vi "CurrentMeterLoop.vi"(8 "Error In":errorcluster, 9 "ABLE Configuration":T1, 10 "Current Meter Data":refnum<notifier>, 11 "Current Meter Action Queue":refnum<queue>) -> (0 "Error Out":errorcluster)   [LabVIEW 2012]
uses:
  CurrentMeterQueueElement.ctl
  CurrentMeterAction.ctl
  ABLEConfiguration.ctl
  DisplayConfiguration.ctl
  FolderConfiguration.ctl
  AlarmsConfiguration.ctl
  Keithley6485Configuration.ctl
  Keithley6482Configuration.ctl
  CurrentMeterData.ctl
  <vilib>/Utility/error.llb/DialogType.ctl
  libs/LV-Utilities/LV-Utilities.lvlib
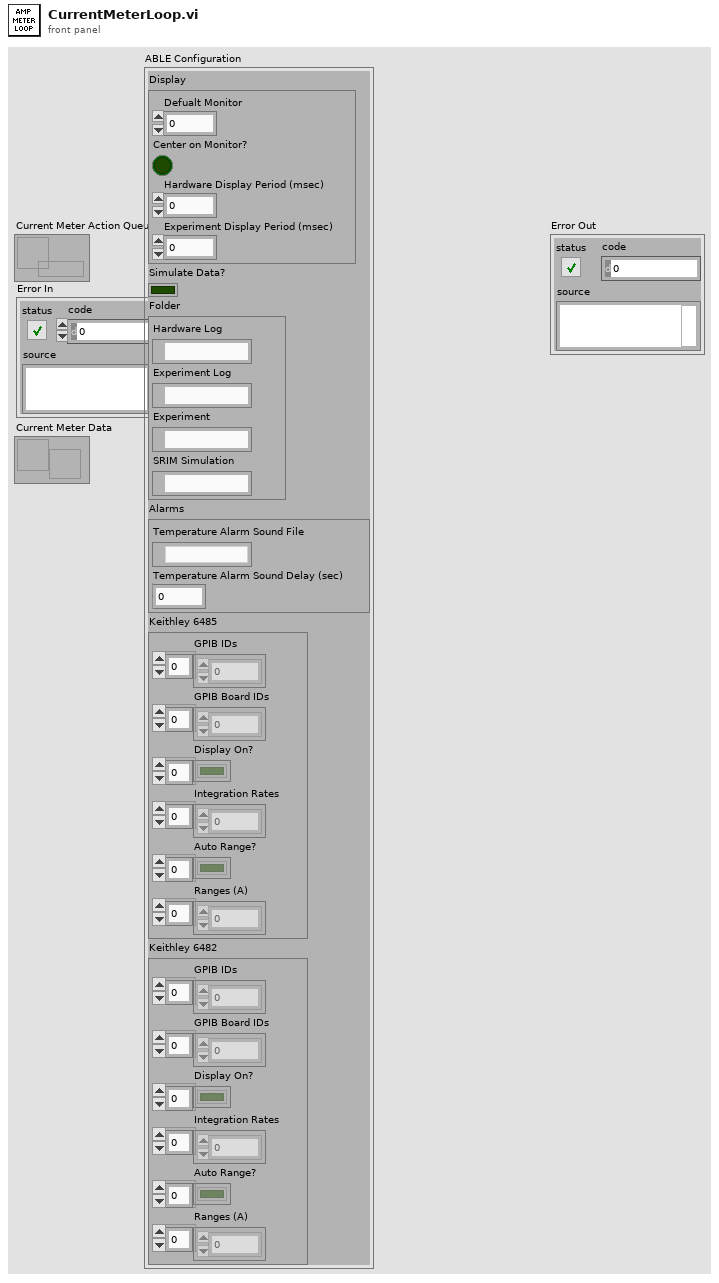
[diagram p1: front panel]
types:
  T1 = typedef "ABLEConfiguration.ctl" = cluster{"Display":T2, "Simulate Data?":bool, "Folder":T3, "Alarms":T4, "Keithley 6485":T5, "Keithley 6482":T6}
  T2 = typedef "DisplayConfiguration.ctl" = cluster{"Defualt Monitor":u16, "Center on Monitor?":bool, "Hardware Display Period (msec)":u32, "Experiment Display Period (msec)":u32}
  T3 = typedef "FolderConfiguration.ctl" = cluster{"Hardware Log":path, "Experiment Log":path, "Experiment":path, "SRIM Simulation":path}
  T4 = typedef "AlarmsConfiguration.ctl" = cluster{"Temperature Alarm Sound File":path, "Temperature Alarm Sound Delay (sec)":dbl}
  T5 = typedef "Keithley6485Configuration.ctl" = cluster{"GPIB IDs":u8[], "GPIB Board IDs":u8[], "Display On?":bool[], "Integration Rates":dbl[], "Auto Range?":bool[], "Ranges (A)":dbl[]}
  T6 = typedef "Keithley6482Configuration.ctl" = cluster{"GPIB IDs":u8[], "GPIB Board IDs":u8[], "Display On?":bool[], "Integration Rates":dbl[], "Auto Range?":bool[], "Ranges (A)":dbl[]}
  T7 = typedef "CurrentMeterData.ctl" = dbl[]
  T8 = typedef "CurrentMeterQueueElement.ctl" = cluster{"Action":T9, "Data":variant}
  T9 = typedef "CurrentMeterAction.ctl" = enum16{"Initialize", "Read", "Simulate", "Error", "Shutdown"}
  T10 = typedef "DialogType.ctl" = u16
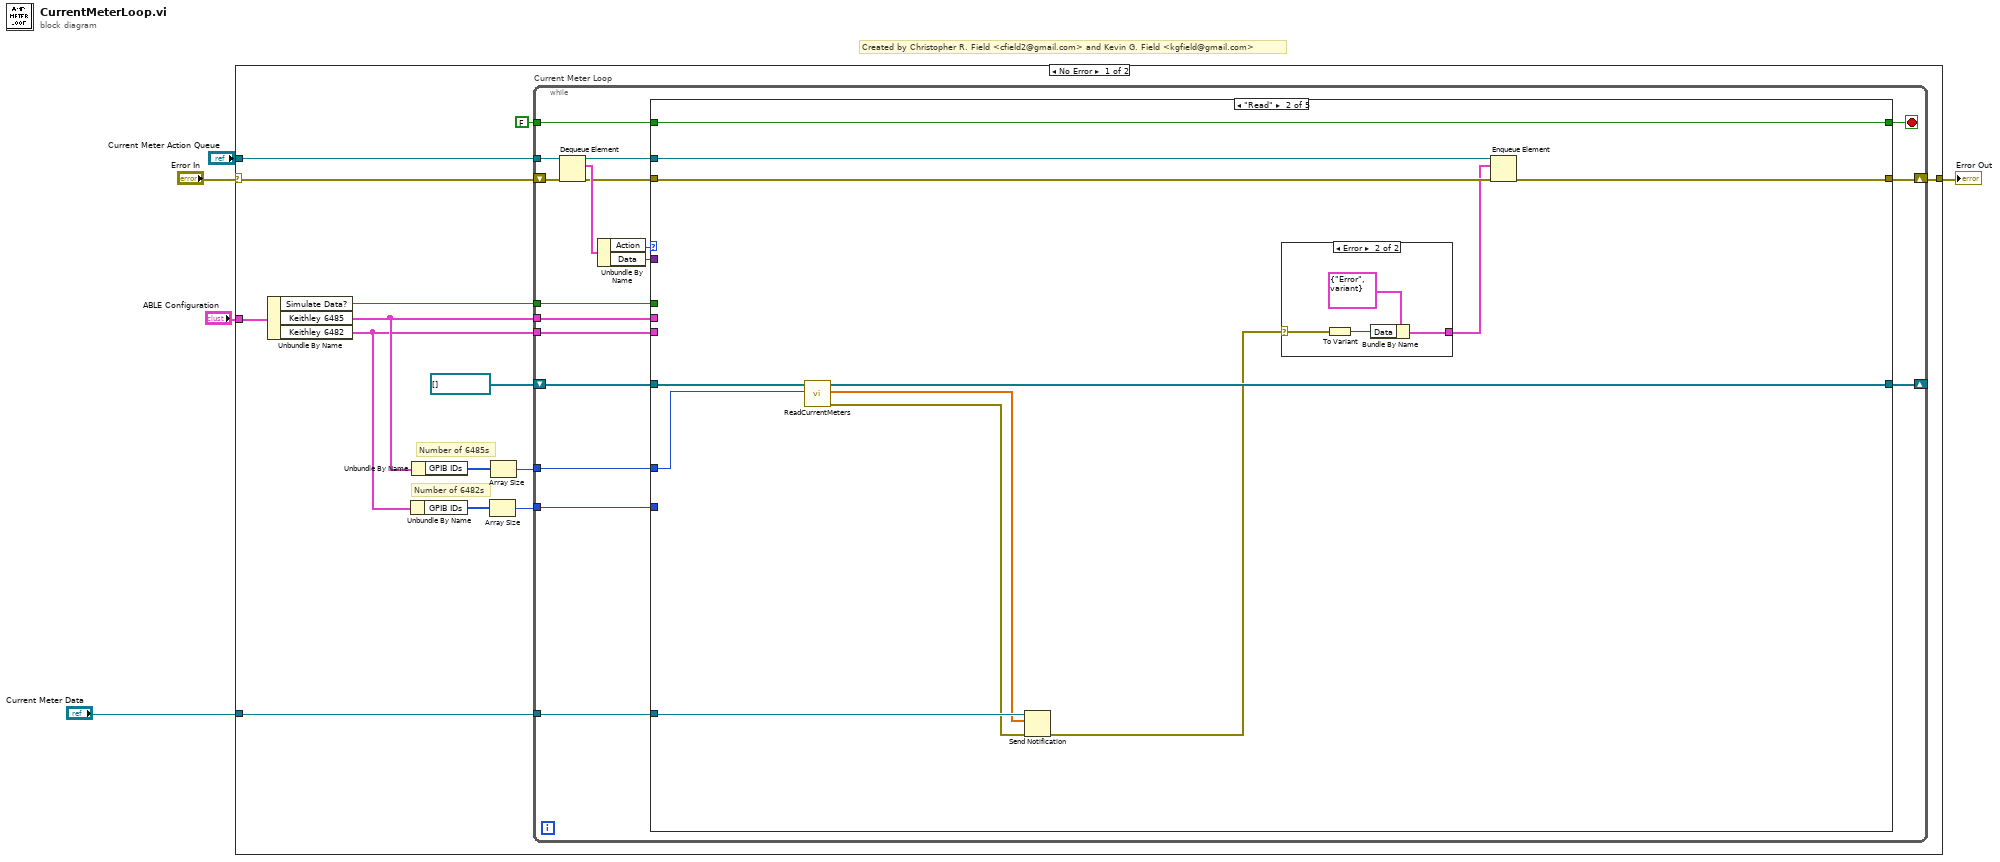
[diagram p0: block diagram]
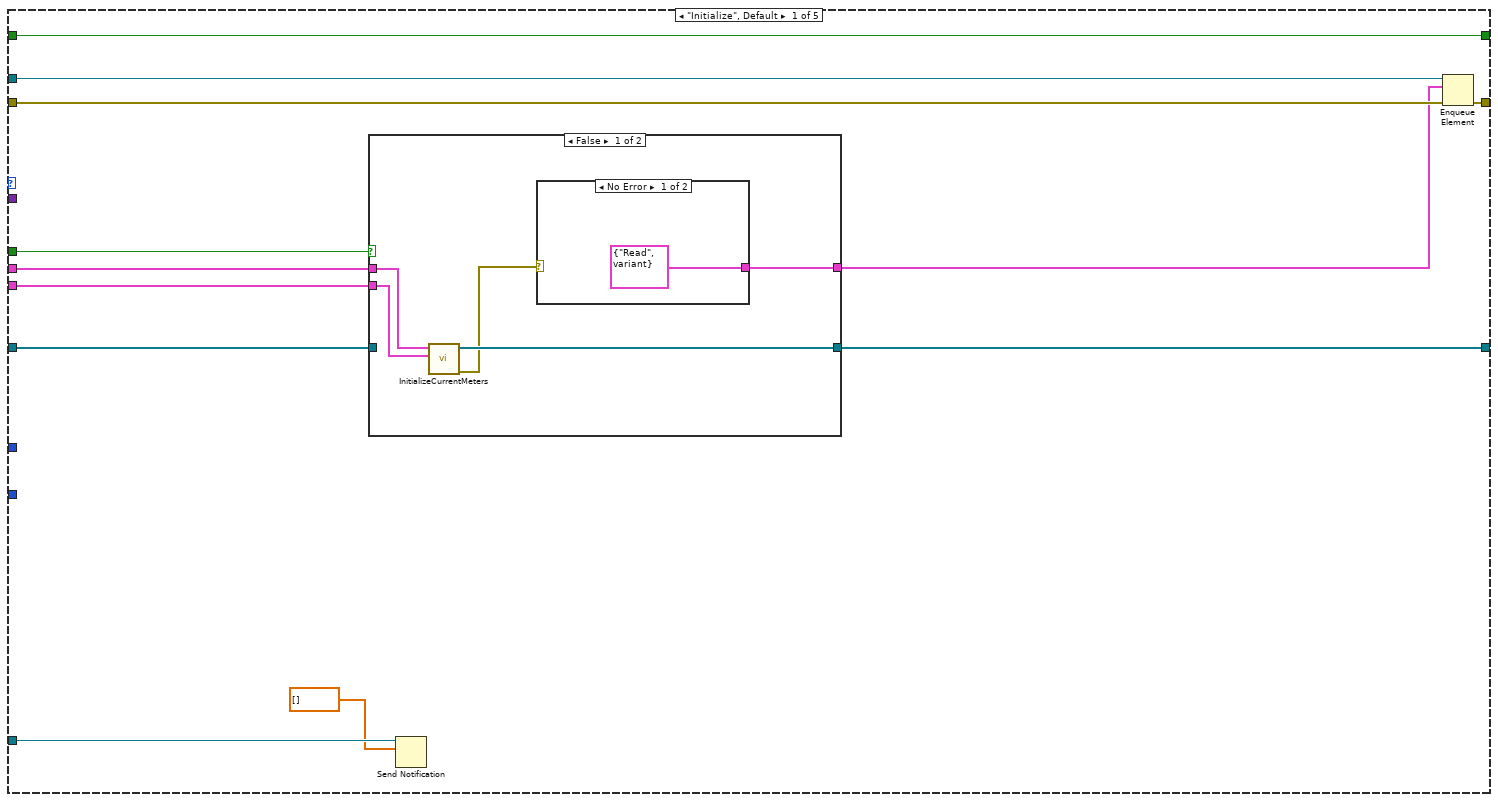
[diagram p2: hidden frame]
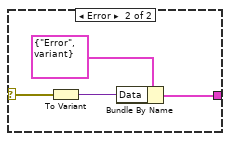
[diagram p3: hidden frame]
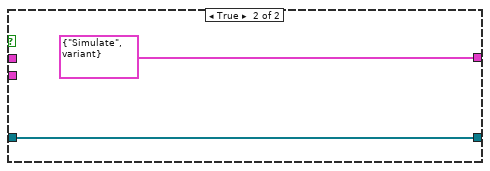
[diagram p4: hidden frame]
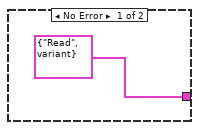
[diagram p5: hidden frame]
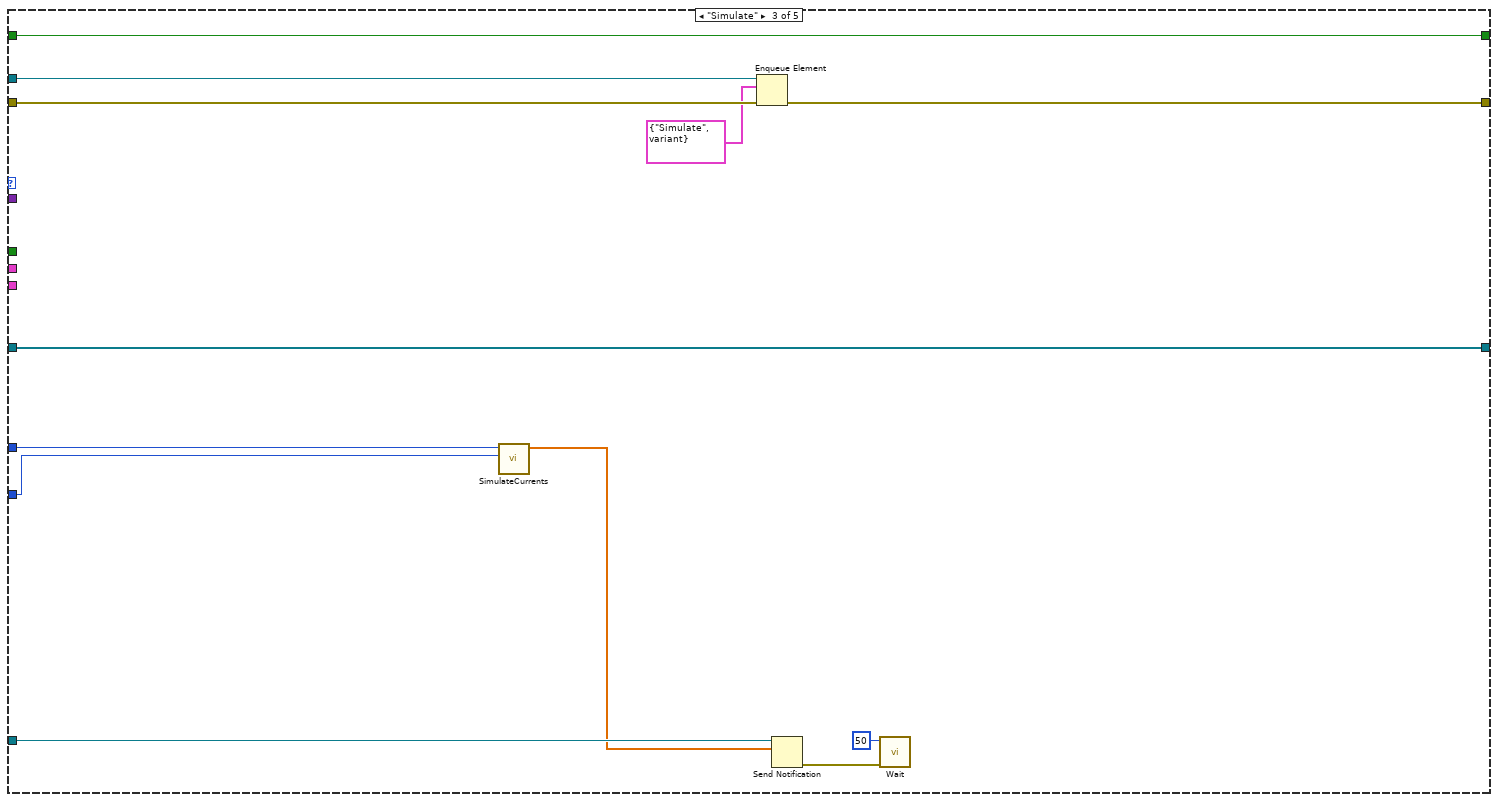
[diagram p6: hidden frame]
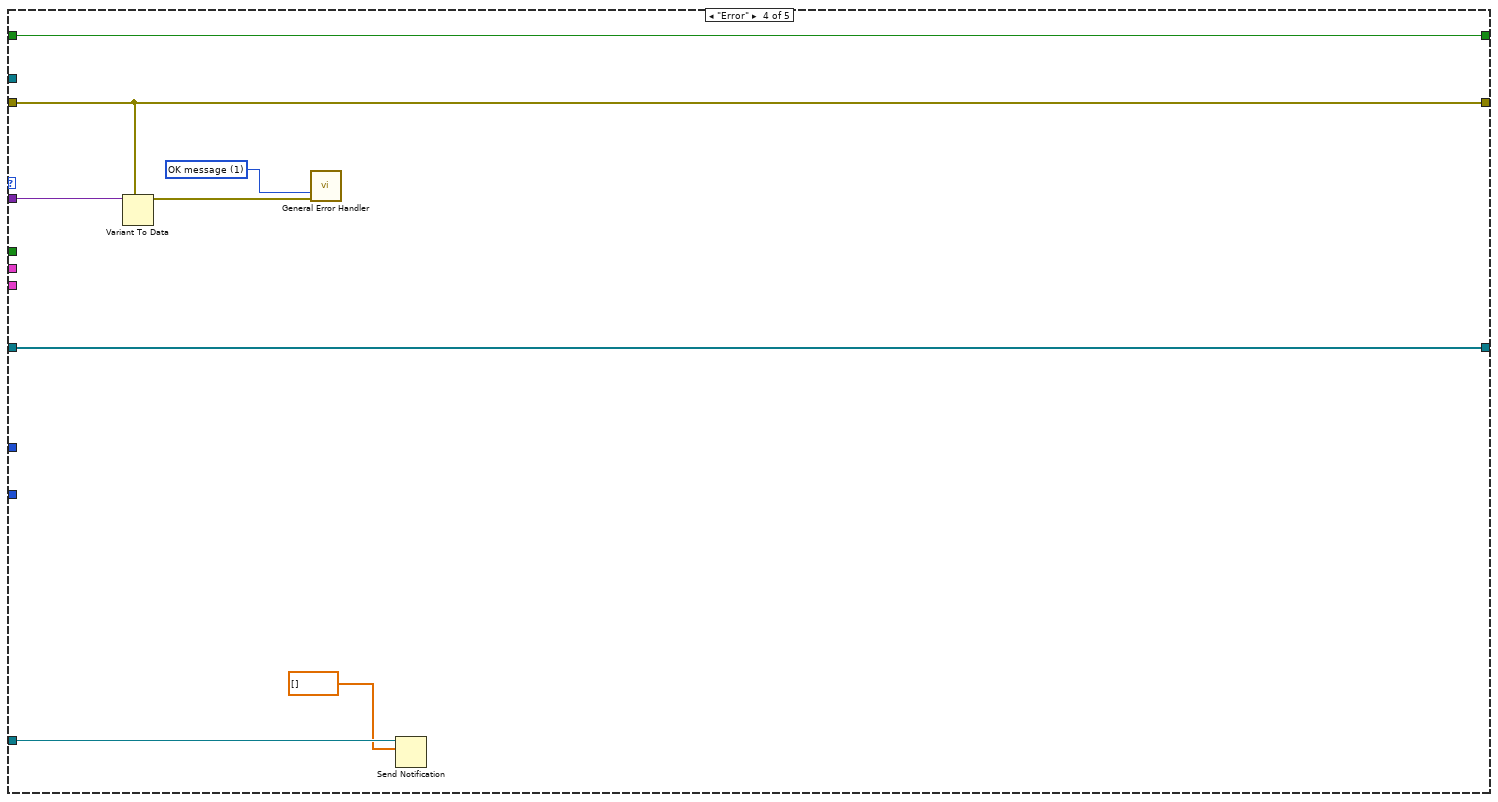
[diagram p7: hidden frame]
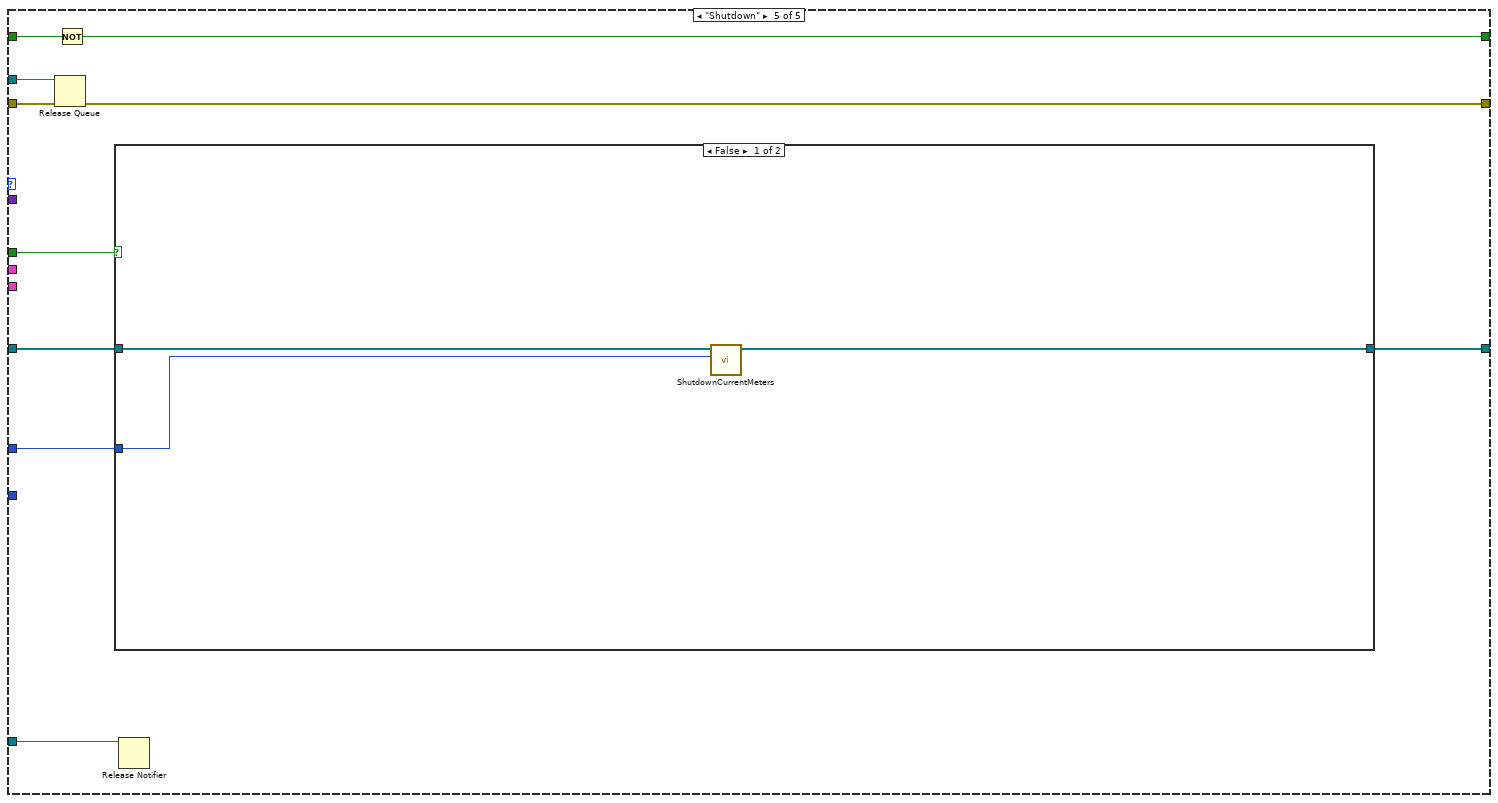
[diagram p8: hidden frame]
diagram:
  # "Created by Christopher R. Field <cfield2@gmail.com> and Kevin G. Field <kgfield@gmail.com>"
  n1 = case shown="No Error" "Error In" {
    selector: "Error In" -> [w17 w113]
    tunnel: "Current Meter Action Queue" -> [w18 _]
    tunnel: [w16 w113] -> w4
    tunnel: "ABLE Configuration" -> [w15 _]
    tunnel: "Current Meter Data" -> [w12 _]
    frame No Error {
      # "Number of 6482s"
      # "Number of 6485s"
      n2 = Unbundle By Name(w15) -> ("Simulate Data?"=w14:bool, "Keithley 6485"=w10:T5, "Keithley 6482"=w7:T6)
      n3 = Unbundle By Name(w7) -> ("GPIB IDs"=w8:u8[])
      n4 = Unbundle By Name(w10) -> ("GPIB IDs"=w11:u8[])
      n5 = Array Size(array=w8) -> (size(s)=w6:i32)
      n6 = Array Size(array=w11) -> (size(s)=w9:i32)
      n7 = while "Current Meter Loop" {
        tunnel: FALSE -> [w35]
        tunnel: w18 -> [w37]
        shift-right: [w28] -> w16
        shift-left: w17 -> [w36]
        tunnel: w14 -> [w27]
        tunnel: w10 -> [w26]
        tunnel: w7 -> [w25]
        shift-right: [w24] -> _
        shift-left: refnum<visa-resource-name>[] [] -> [w23]
        tunnel: w12 -> [w22]
        tunnel: w9 -> [w21]
        tunnel: w6 -> [w20]
        stop <- w29 stop-if-true
        n8 = Dequeue Element(queue=w37, error in (no error)=w36) -> (queue out=w31:refnum<queue>, element=w34:T8, error out=w30:errorcluster)  [unwired: 1 in, 1 out]
        n9 = Unbundle By Name(w34) -> ("Action"=w33:T9, "Data"=w32:variant)
        n10 = case shown="\"Read\"" w33 {
          tunnel: w35 -> [w49 w73 w90 w98 w108]
          tunnel: w32 -> [_ _ _ w97 _]
          tunnel: w31 -> [w48 w72 w89 _ w106]
          tunnel: w30 -> [w47 w71 w88 w96 w105]
          tunnel: [w49 w73 w90 w98 w107] -> w29
          tunnel: [w46 w70 w87 w96 w104] -> w28
          tunnel: w27 -> [w45 _ _ _ w103]
          tunnel: w26 -> [w43 _ _ _ _]
          tunnel: w25 -> [w42 _ _ _ _]
          tunnel: [w41 w67 w83 w93 w101] -> w24
          tunnel: w23 -> [w40 w68 w83 w93 w102]
          tunnel: w22 -> [w39 w65 w82 w92 w100]
          tunnel: w21 -> [_ w63 w80 _ w99]
          tunnel: w20 -> [_ _ w79 _ _]
          frame "Initialize", Default {
            n11 = case shown="False" w45 {
              tunnel: [w54 T8 {"Action"=enum."Simulate", "Data"=variant} ("element")] -> w44
              tunnel: w43 -> [w53 _]
              tunnel: w42 -> [w52 _]
              tunnel: [w51 w60] -> w41
              tunnel: w40 -> [_ w60]
              frame False {
                n12 = call "InitializeCurrentMeters.vi"("Keithley 6482"=w52, "Keithley 6485"=w53) -> ("Error Out"=w50:errorcluster, "Current Meters Out"=w51:refnum<visa-resource-name>[])  [unwired: 8 in]
                n13 = case shown="No Error" w50 {
                  selector: w50 -> [_ w58]
                  tunnel: [T8 {"Action"=enum."Read", "Data"=variant} ("element") w56] -> w54
                  frame No Error {
                  }
                  frame Error {
                    n14 = To Variant(anything=w58) -> (Variant=w57:variant)
                    n15 = Bundle By Name(cluster=T8 {"Action"=enum."Error", "Data"=variant} ("element"), "Data"=w57) -> (w56:T8)
                  }
                }
              }
              frame True {
              }
            }
            n16 = Send Notification(notification=T7 [], notifier=w39) -> ()  [unwired: 1 in, 2 out]
            n17 = Enqueue Element(queue=w48, element=w44, error in (no error)=w47) -> (error out=w46:errorcluster)  [unwired: 1 in, 2 out]
          }
          frame "Read" {
            n18 = call "ReadCurrentMeters.vi"("Number of 6485"=w63, "Current Meters In"=w68) -> ("Error Out"=w62:errorcluster, "Current Meter Data"=w64:T7, "Current Meters Out"=w67:refnum<visa-resource-name>[])  [unwired: 7 in]
            n19 = Send Notification(notification=w64, notifier=w65, error in (no error)=w62) -> (error out=w66:errorcluster)  [unwired: 1 out]
            n20 = case shown="Error" w66 {
              selector: w66 -> [_ w75]
              tunnel: [T8 {"Action"=enum."Read", "Data"=variant} ("element") w77] -> w69
              frame No Error {
              }
              frame Error {
                n21 = To Variant(anything=w75) -> (Variant=w76:variant)
                n22 = Bundle By Name(cluster=T8 {"Action"=enum."Error", "Data"=variant} ("element"), "Data"=w76) -> (w77:T8)
              }
            }
            n23 = Enqueue Element(queue=w72, element=w69, error in (no error)=w71) -> (error out=w70:errorcluster)  [unwired: 1 in, 2 out]
          }
          frame "Simulate" {
            n24 = call "SimulateCurrents.vi"("Number of 6482s"=w79, "Number of 6485s"=w80) -> ("Current Meter Data"=w81:T7)  [unwired: 9 in]
            n25 = Enqueue Element(queue=w89, element=T8 {"Action"=enum."Simulate", "Data"=variant}, error in (no error)=w88) -> (error out=w87:errorcluster)  [unwired: 1 in, 2 out]
            n26 = Send Notification(notification=w81, notifier=w82) -> (error out=w85:errorcluster)  [unwired: 1 in, 1 out]
            n27 = call "Wait.vi"("Error In"=w85, "Wait Time (msec)"=u32 50) -> ()  [unwired: 9 in, 1 out]
          }
          frame "Error" {
            w94 = T10 1 items=["no dialog", "OK message", "continue or stop message", "OK message + warnings", "continue/stop + warnings"] ("type of dialog (OK msg:1)")
            n28 = Variant To Data(type=w96, Variant=w97) -> (data=w95:errorcluster)  [unwired: 1 in, 1 out]
            n29 = call <vilib>:"General Error Handler.vi"("type of dialog (OK msg:1)"=w94, "error in (no error)"=w95) -> ()  [unwired: 9 in, 5 out]
            n30 = Send Notification(notification=T7 [], notifier=w92) -> ()  [unwired: 1 in, 2 out]
          }
          frame "Shutdown" {
            n31 = Release Queue(queue=w106, error in (no error)=w105) -> (error out=w104:errorcluster)  [unwired: 1 in, 2 out]
            n32 = Not(x=w108) -> (.not. x?=w107:bool)
            n33 = case shown="False" w103 {
              tunnel: w102 -> [w111 w112]
              tunnel: [w110 w112] -> w101
              tunnel: w99 -> [w109 _]
              frame False {
                n34 = call "ShutdownCurrentMeters.vi"("Number of 6485s"=w109, "Current Meters In"=w111) -> ("Current Meters Out"=w110:refnum<visa-resource-name>[])  [unwired: 8 in, 1 out]
              }
              frame True {
              }
            }
            n35 = Release Notifier(notifier=w100) -> ()  [unwired: 2 in, 3 out]
          }
        }
      }
    }
    frame Error {
    }
  }
  "Error Out" <- w4
